vi "PH_Beckhoff_Application.declare digital MA01 InputTags.vi"() -> (0 "Digital Inputs":T2, 1 "Description":string)   [LabVIEW 2014, in "PH_Beckhoff_Application.lvlib"]
uses:
  PH_Beckhoff_Application.lvlib
  PH_Beckhoff/PH_Beckhoff.Digital Inputs.ctl
  PH_Beckhoff/PH_Beckhoff.lvlib
panel:
  in  "Digital Input Value":T1
  out "Right Size?":bool
  # "Let this VI run to check the size!"
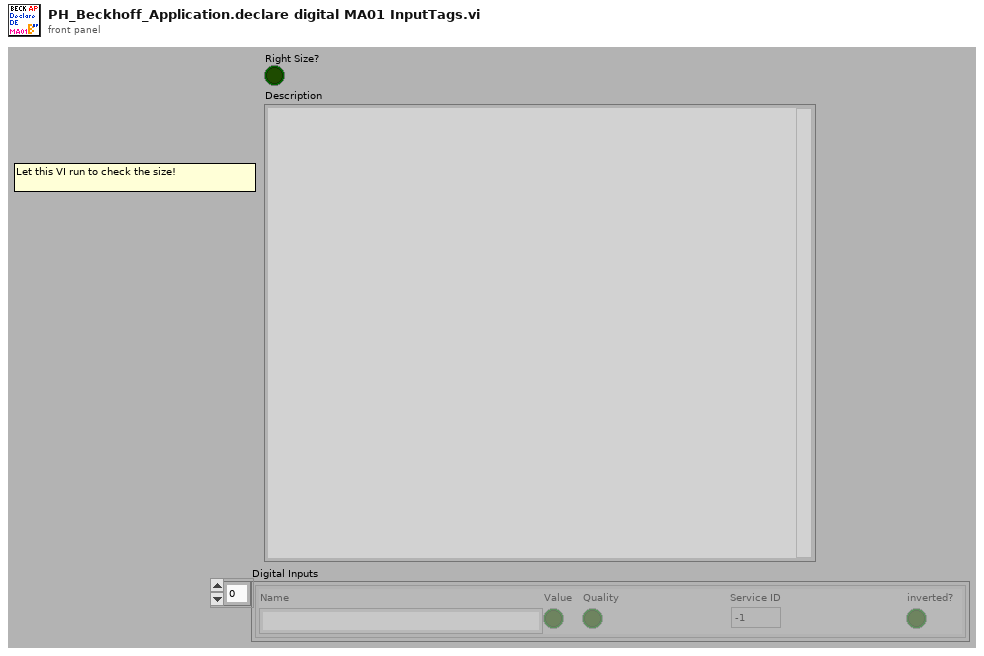
[diagram p1: front panel]
types:
  T1 = cluster{"Name":string, "Value":bool, "Quality":bool, "Service ID":i32, "inverted?":bool}
  T2 = typedef "PH_Beckhoff.lvlib/PH_Beckhoff.Digital Inputs.ctl" = cluster{"Name":string, "Value":bool, "Quality":bool, "Service ID":i32, "inverted?":bool}[]
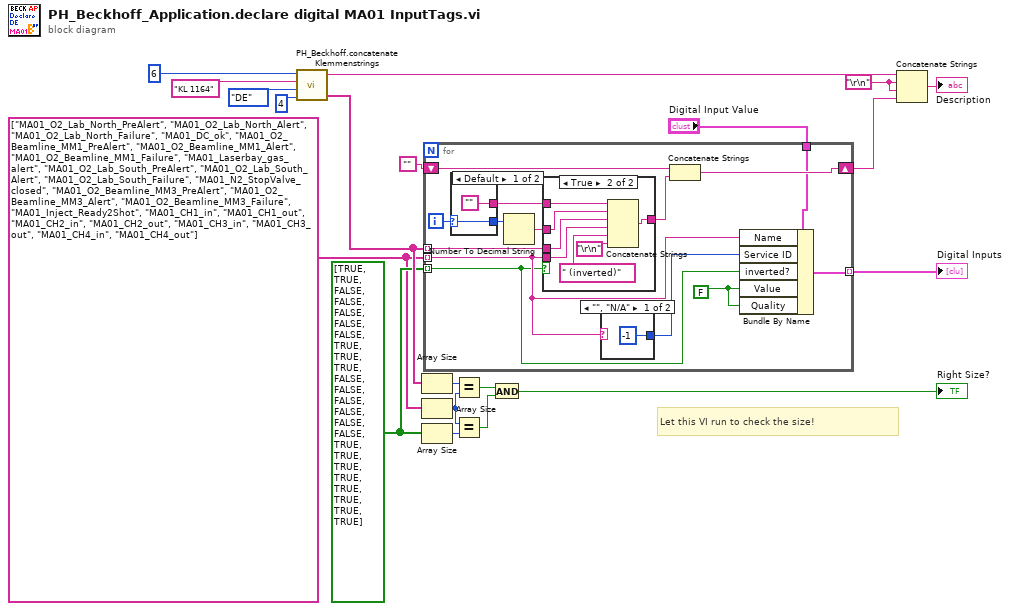
[diagram p0: block diagram]
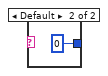
[diagram p2: hidden frame]
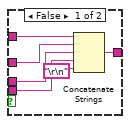
[diagram p3: hidden frame]
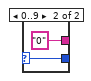
[diagram p4: hidden frame]
diagram:
  w4 = bool[] [TRUE, TRUE, FALSE, FALSE, FALSE, FALSE, FALSE, TRUE, TRUE, TRUE, FALSE, FALSE, FALSE, FALSE, FALSE, FALSE, TRUE, TRUE, TRUE, TRUE, TRUE, TRUE, TRUE, TRUE]
  w3 = string[] ["MA01_O2_Lab_North_PreAlert", "MA01_O2_Lab_North_Alert", "MA01_O2_Lab_North_Failure", "MA01_DC_ok", "MA01_O2_Beamline_MM1_PreAlert", "MA01_O2_Beamline_MM1_Alert", "MA01_O2_Beamline_MM1_Failure", "MA01_Laserbay_gas_alert", "MA01_O2_Lab_South_PreAlert", "MA01_O2_Lab_South_Alert", "MA01_O2_Lab_South_Failure", "MA01_N2_StopValve_closed", "MA01_O2_Beamline_MM3_PreAlert", "MA01_O2_Beamline_MM3_Alert", "MA01_O2_Beamline_MM3_Failure", "MA01_Inject_Ready2Shot", "MA01_CH1_in", "MA01_CH1_out", "MA01_CH2_in", "MA01_CH2_out", "MA01_CH3_in", "MA01_CH3_out", "MA01_CH4_in", "MA01_CH4_out"]
  w18 = "\r\n"
  # "Let this VI run to check the size!"
  n1 = call "PH_Beckhoff.concatenate Klemmenstrings.vi"("# of In- or Outputs"=4, "Type"=enum16{"AE", "AA", "DE", "DA"}."DE", "Klemmenname"="KL 1164", "Quantity"=6) -> ("concatenated string array"=w10:string[], "\"<Type>: <Quantity> x <Klemmenname>\""=w11:string)  [unwired: 1 out]
  n2 = Array Size(array=w10) -> (size(s)=w16:i32)
  n3 = Array Size(array=w3) -> (size(s)=w9:i32)
  n4 = Array Size(array=w4) -> (size(s)=w8:i32)
  n5 = for {
    tunnel: w3 -> [w25] mode=indexing
    tunnel: w10 -> [w30] mode=indexing
    shift-right: [w28] -> w19
    shift-left: "" -> [w27]
    tunnel: w4 -> [w23] mode=indexing
    tunnel: "Digital Input Value" -> [w26]
    tunnel: [w21] -> w1 mode=indexing
    i -> [w34]
    w22 = FALSE ("Quality")
    n6 = case shown="Default" w34 {
      selector: w34 -> [w50 w53]
      tunnel: [w50 w53] -> w33
      tunnel: ["" "0"] -> w32
      frame Default {
      }
      frame 0..9 {
      }
    }
    n7 = Number To Decimal String(number=w33) -> (decimal integer string=w31:string)  [unwired: 1 in]
    n8 = case shown="True" w23 {
      tunnel: w32 -> [w42 w49]
      tunnel: w31 -> [w41 w48]
      tunnel: w30 -> [w40 w47]
      tunnel: w25 -> [w39 w46]
      tunnel: [w37 w44] -> w29
      frame False {
        n9 = Concatenate Strings(w42, w41, w40, w39, "\r\n") -> (w37:string)
      }
      frame True {
        n10 = Concatenate Strings(w49, w48, w47, w46, " (inverted)" ("string"), "\r\n") -> (w44:string)
      }
    }
    n11 = case shown="\"\", \"N/A\"" w25 {
      tunnel: [-1 0] -> w24
      frame "", "N/A" {
      }
      frame Default {
      }
    }
    n12 = Concatenate Strings(w27, w29) -> (w28:string)
    n13 = Bundle By Name(cluster=w26, "Name"=w25, "Service ID"=w24, "inverted?"=w23, "Value"=w22, "Quality"=w22) -> (w21:T1)
  }
  "Digital Inputs" <- w1
  n14 = Equal?(x=w16, y=w9) -> (x = y?=w6:bool)
  n15 = Equal?(x=w9, y=w8) -> (x = y?=w5:bool)
  n16 = And(x=w6, y=w5) -> (x .and. y?=→"Right Size?":bool)
  n17 = Concatenate Strings(w11, w18, w18, w19) -> (→"Description":string)
